vi "FPPublisher.vi"   [LabVIEW 2014]
uses:
  WebFrontPanel_class/WebFrontPanel.lvclass
  FrontPanelManager_class/FrontPanelManager.lvclass
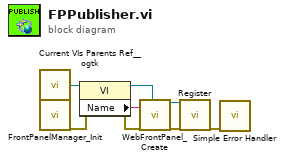
[diagram p0: block diagram]
diagram:
  n1 = call <userlib>:"Current VIs Parents Ref__ogtk.vi"() -> ("Calling VI's Reference"=w5:refnum<vi>)  [unwired: 2 in]
  n2 = call "FrontPanelManager_Init.vi"() -> ("error out"=w3:errorcluster)  [unwired: 18 in, 1 out]
  n3 = property class="VI"(reference=w5, error in=w3) -> (reference out=w4:refnum<vi>, error out=w2:errorcluster, "Name"=w8:string)
  n4 = call "WebFrontPanel_Create.vi"("VI Name"=w8, "error in (no error)"=w2, "VI Reference"=w4) -> ("reference out"=w6:refnum<class "WebFrontPanel.lvclass">, "error out"=w7:errorcluster)  [unwired: 15 in]
  n5 = call "Register.vi"("WebFrontPanel"=w6, "error in (no error)"=w7) -> ("error out"=w1:errorcluster)  [unwired: 17 in]
  n6 = call <vilib>:"Simple Error Handler.vi"("error in (no error)"=w1) -> ()  [unwired: 4 in, 5 out]
